vi "Init.vi"(8 "error in (no error)":errorcluster, 11 "VISA resource name":refnum<visa-resource-name>) -> (0 "error out":errorcluster, 2 "Instrument Identification":string, 3 "VISA resource name out":refnum<visa-resource-name>)   [LabVIEW 2023, in "Keysight-34450A.lvlib"]
doc: "<b>Author:</b> Wolfgang\n<b>Description:</b> Initializes the instrument Reference"
uses:
  Keysight-34450A.lvlib
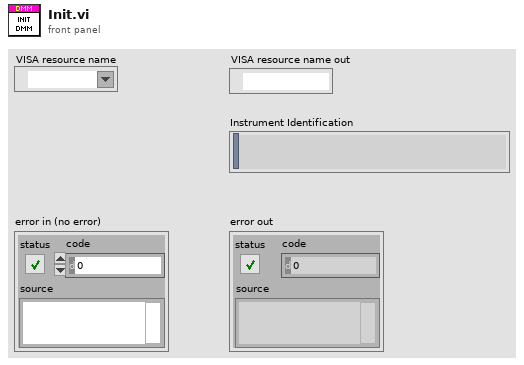
[diagram p1: front panel]
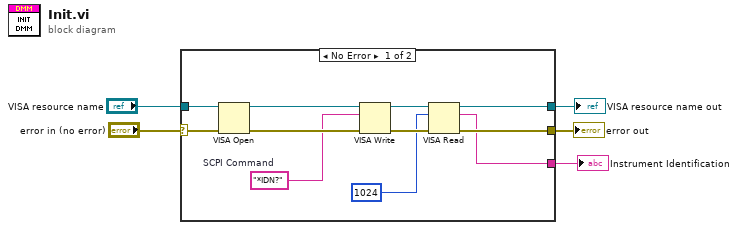
[diagram p0: block diagram]
diagram:
  n1 = case shown="No Error" "error in (no error)" {
    selector: "error in (no error)" -> [w8 w18]
    tunnel: [w16 w17] -> w5
    tunnel: [w14 w18] -> w3
    tunnel: "VISA resource name" -> [w9 w17]
    tunnel: [w12 _] -> w1
    frame No Error {
      w6 = "*IDN?"  # SCPI Command
      n2 = VISA Open(error in (no error)=w8, VISA resource name=w9) -> (VISA resource name=w10:refnum<visa-resource-name>, error out=w7:errorcluster)  [unwired: 3 in]
      n3 = VISA Write(VISA resource name=w10, write buffer=w6, error in (no error)=w7) -> (VISA resource name out=w13:refnum<visa-resource-name>, error out=w15:errorcluster)  [unwired: 1 out]
      n4 = VISA Read(VISA resource name=w13, byte count=u32 1024, error in (no error)=w15) -> (VISA resource name out=w16:refnum<visa-resource-name>, read buffer=w12:string, error out=w14:errorcluster)  [unwired: 1 out]
    }
    frame Error {
    }
  }
  "VISA resource name out" <- w5
  "error out" <- w3
  "Instrument Identification" <- w1
